vi "Untitled 1.vi"   [LabVIEW 2013]
uses:
  C:/Program Files/Princeton Instruments/LightField/PrincetonInstruments.LightFieldAddInSupportServices.dll
  Program Files/Princeton Instruments/LightField/PrincetonInstruments.LightFieldAddInSupportServices.dll
  lightfield-automation-labview/VIs/ClientServerMode/CS_LFAClassGlobal.vi
  lightfield-automation-labview/LightField Automation.lvclass
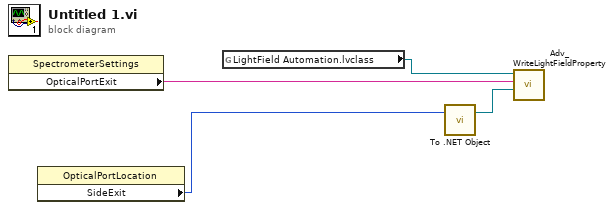
[diagram p0: block diagram]
diagram:
  n1 = property class="SpectrometerSettings"() -> ("OpticalPortExit"=w3:string)  [unwired: 2 in, 2 out]
  n2 = property class="OpticalPortLocation"() -> ("SideExit"=w1:i32)  [unwired: 2 in, 2 out]
  n3 = global read "CS_LFAClassGlobal.vi" "LightField Automation.lvclass"() -> (w4:refnum<class "LightField Automation.lvclass">)
  n4 = call <vilib>:"To .NET Object.vi"("anything"=w1) -> (".NET object"=w2:refnum<k24>)  [unwired: 1 in, 1 out]
  n5 = call "Adv_WriteLightFieldProperty.vi"("value"=w2, "setting"=w3, "LightField Automation in"=w4) -> ()  [unwired: 7 in, 2 out]
